vi "TestExec.Set Mode Control Color.vi"(8 "error in":errorcluster, 9 "Mode Config":cluster{"Name":string, "Color":u32}[](array[cluster])=[{"Name"="Production", "Color"=15204328}, {"Name"="Technician", "Color"=16383928}, {"Name"="Engineering", "Color"=13629951}, {"Name"="Maintenance", "Color"=16764882}, {"Name"="Validation", "Color"=15376639}], 11 "Mode Control":refnum<vi>) -> (0 "error out":errorcluster)   [LabVIEW 2018]
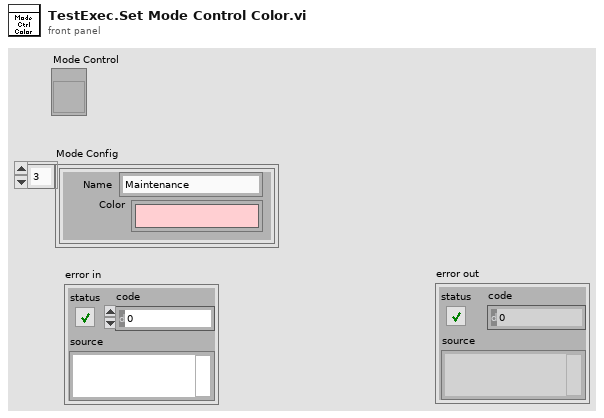
[diagram p1: front panel]
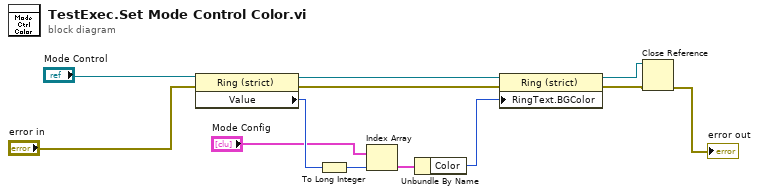
[diagram p0: block diagram]
diagram:
  n1 = property class="Ring (strict)"(reference="Mode Control", error in="error in") -> (reference out=w5:refnum<vi>, error out=w6:errorcluster, "Value"=w11:u16)
  n2 = To Long Integer(number=w11) -> (32bit integer=w10:i32)
  n3 = Index Array(array="Mode Config", index=w10) -> (element=w9:cluster{"Name":string, "Color":u32})
  n4 = Unbundle By Name(w9) -> ("Color"=w8:u32)
  n5 = property class="Ring (strict)"(reference=w5, error in=w6, "RingText.BGColor"=w8) -> (reference out=w2:refnum<vi>, error out=w4:errorcluster)
  n6 = Close Reference(reference=w2, error in (no error)=w4) -> (error out=→"error out":errorcluster)
